vi "PH_PILS.PC _SpecialBoolean.vi"(0 "i ref in":refnum<vi>, 2 "serviceName":string, 3 "Value":i32, 5 "error IO":errorcluster) -> (14 "i ref out":refnum<vi>, 19 "error out":errorcluster)   [LabVIEW 2014, in "PH_PILS.lvlib"]
doc: "This is the proc case \"_SpecialBoolean\"."
uses:
  PH_PILS.lvlib
  PH_Basics/PH_Common/PH_Common.lvlib
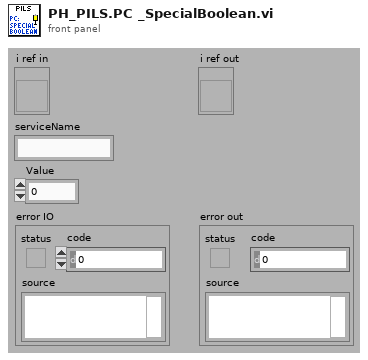
[diagram p1: front panel]
types:
  T1 = typedef "PH_PILS.lvlib/PH_PILS.i attribute.ctl" = cluster{"Boolean":cluster{"GUI Ref":refnum<vi>, "Status":i32}[], "GUI Refs Exp. Shutters":cluster{"1":refnum<vi>, "2":refnum<vi>, "3":refnum<vi>, "4":refnum<vi>}, "Tristate2Run GUI Refs":refnum<vi>[], "EO-Likes":cluster{"GUI Ref":refnum<vi>, "Status":i32}[], "Operation Mode":cluster{"Operation Mode":T2, "GUI":cluster{"Ref State":refnum<vi>, "Ref":refnum<vi>}, "Servicemode":cluster{"Tagname":string, "Status":i32}, "Labormode":cluster{"Tagname":string, "Status":i32}, "Searchmode":cluster{"Tagname":string, "Status":i32}, "Shotmode":cluster{"Tagname":string, "Status":i32}}, "Submode":cluster{"Submode":T3, "GUI":cluster{"Ref State":refnum<vi>, "Ref":refnum<vi>}, "Submode":cluster{"Tagname":string, "Status":i32}}, "Experiment":cluster{"Experiment":enum16{"unknown", "intern", "4 (Z6)", "3", "2", "1"}, "GUI":cluster{"Ref State":refnum<vi>, "Ref":refnum<vi>}, "intern":cluster{"Tagname":string, "Status":i32}, "Exp 4":cluster{"Tagname":string, "Status":i32}, "Exp 3":cluster{"Tagname":string, "Status":i32}, "Exp 2":cluster{"Tagname":string, "Status":i32}, "Exp 1":cluster{"Tagname":string, "Status":i32}}, "TristateNormal":cluster{"GUI Ref":refnum<vi>, "Status":i32}[], "Door Tags":cluster{"GUI Ref":refnum<vi>, "Status":i32}[], "GUIlessTags":cluster{"Name":string, "Status":i32}[], "Beamline GUI Refs":refnum<vi>[], "Special Boolean":cluster{"GUI Ref":refnum<vi>, "Status":i32}[], "Laserpower":cluster{"GUI Ref":refnum<vi>, "Status":i32}[], "Shutter":cluster{"GUI Ref":refnum<vi>, "Status":i32}[], "Tristate EO Like":cluster{"GUI Ref":refnum<vi>, "Status":i32}[], "PP":cluster{"GUI Ref":refnum<vi>, "Status":i32, "Head Ref":refnum<vi>, "Slider Ref":refnum<vi>}[], "Switch Knobs":cluster{"GUI Ref":refnum<vi>, "Status":i32}[], "Latch Knob GUI Refs":refnum<vi>[], "FailureCounter":i32, "Enabled Status":cluster{"Laser":i32, "PreAmp":i32, "MainAmp":i32}, "Mercury":refnum<vi>, "Instance Rods":string, "Logfile":path, "Beckhoff-Instance Internal":string, "Beckhoff-Instance External":string, "Enabling Rights":cluster{"Name":string, "Password":string, "PA?":bool, "MA?":bool, "Exp?":bool}[]}
  T2 = typedef "PH_PILS.lvlib/PH_PILS.Operation Mode.ctl" = enum16{"unknown", "Service", "Labor", "Search", "Shot"}
  T3 = typedef "PH_PILS.lvlib/PH_PILS.Submode.ctl" = enum16{"unknown", "HV-Normal", "HV-Test"}
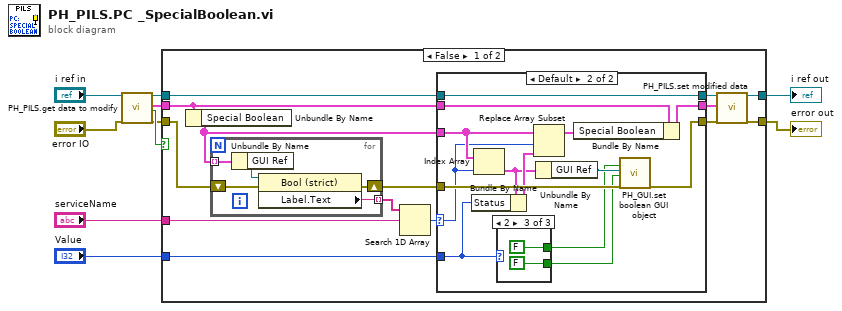
[diagram p0: block diagram]
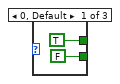
[diagram p3: hidden frame]
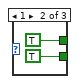
[diagram p4: hidden frame]
diagram:
  n1 = call "PH_PILS.get data to modify.vi"("i ref in"="i ref in", "error in (no error)"="error IO") -> ("i ref out"=w5:refnum<vi>, "i attribute"=w8:T1, "timed out"=w10:bool, "error out"=w6:errorcluster)  [unwired: 14 in]
  n2 = case shown="False" w10 {
    tunnel: w5 -> [w24 w54]
    tunnel: [w12 w54] -> w2
    tunnel: [w15 w53] -> w1
    tunnel: w6 -> [w23 w53]
    tunnel: "serviceName" -> [w20 _]
    tunnel: w8 -> [w17 _]
    tunnel: "Value" -> [w16 _]
    frame False {
      n3 = Unbundle By Name(w17) -> ("Special Boolean"=w18:cluster{"GUI Ref":refnum<vi>, "Status":i32}[])
      n4 = for {
        tunnel: w18 -> [w50] mode=indexing
        shift-right: [w52] -> w22
        shift-left: w23 -> [w51]
        tunnel: [w48] -> w21 mode=indexing
        n5 = Unbundle By Name(w50) -> ("GUI Ref"=w49:refnum<vi>)
        n6 = property class="Bool (strict)"(reference=w49, error in=w51) -> (error out=w52:errorcluster, "Label.Text"=w48:string)  [unwired: 1 out]
      }
      n7 = Search 1D Array(1D array=w21, element=w20) -> (index of element=w19:i32)  [unwired: 1 in]
      n8 = case shown="Default" w19 {
        selector: w19 -> [_ w34]
        tunnel: w24 -> [w27 w33]
        tunnel: [w27 w33] -> w13
        tunnel: [w26 w32] -> w14
        tunnel: w22 -> [w26 w39]
        tunnel: w18 -> [_ w40]
        tunnel: w17 -> [w25 w38]
        tunnel: w16 -> [_ w30]
        tunnel: [w25 w31] -> w11
        frame -1 {
        }
        frame Default {
          n9 = Index Array(array=w40, index=w34) -> (element=w35:cluster{"GUI Ref":refnum<vi>, "Status":i32})
          n10 = Bundle By Name(cluster=w35, "Status"=w30) -> (w37:cluster{"GUI Ref":refnum<vi>, "Status":i32})
          n11 = case shown="2" w30 {
            tunnel: [TRUE ("Visible (true)") TRUE ("Visible (true)") FALSE ("Visible (true)")] -> w29
            tunnel: [FALSE TRUE FALSE] -> w28
            frame 0, Default {
            }
            frame 1 {
            }
            frame 2 {
            }
          }
          n12 = Replace Array Subset(array=w40, new element=w37, index=w34) -> (w41:cluster{"GUI Ref":refnum<vi>, "Status":i32}[])
          n13 = Unbundle By Name(w35) -> ("GUI Ref"=w36:refnum<vi>)
          n14 = Bundle By Name(cluster=w38, "Special Boolean"=w41) -> (w31:T1)
          n15 = call "PH_GUI.set boolean GUI object.vi"("Visible (true)"=w29, "Boolean Knob GUI Ref"=w36, "Value"=w28, "error in (no error)"=w39) -> ("error out"=w32:errorcluster)  [unwired: 15 in]
        }
      }
      n16 = call "PH_PILS.set modified data.vi"("i ref in"=w13, "i attribute"=w11, "error in (no error)"=w14) -> ("i ref out"=w12:refnum<vi>, "error out"=w15:errorcluster)  [unwired: 15 in]
    }
    frame True {
    }
  }
  "error out" <- w1
  "i ref out" <- w2
